vi "Send string and wait for answer or timeout.vi"(0 "System no.":i32=1 min=1 max=4 step=1, 2 "String to send":string, 3 "Attach Linefeed?":bool=TRUE, 4 "Timeout, sec":u32=60, 5 "error in":errorcluster, 12 "Stop refnum":refnum<vi>) -> (14 "String read":string, 15 "Stopped?":bool, 19 "error out":errorcluster)   [LabVIEW 2026]
doc: "Sends a string and waits until an answer has come or a timeout-condition has occured. Timeout is independent of the global communication timeout value. Sends #24 if VI was stopped. Needed by INI hexaxes and wait until finished.vi.\n\nC-887, F-206, M-8X0: INI procedure of GCS 1.0 firmware (Check with CSV?.vi. If CSV?.vi is not supported, syntax version is GCS 1.0) can be stopped with #24 since firmware version 4.0.0 (F-206) and 4.5.0 (M-8X0)."
uses:
  Communication/Global1.vi
panel:
  in  "Local stop":bool
  # "Sends a string and waits until an answer has come, a timeout \ncondition has occured, Local stop is TRUE or Stop refnum is TRUE.\n\"Timeout\" is independent of the global communication timeout \nvalue. Needed by \"INI hexaxes and wait until finished.vi\"."
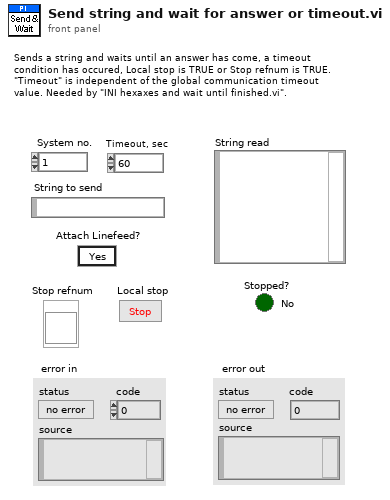
[diagram p1: front panel]
types:
  T1 = typedef "Semaphore RefNum" = refnum<k1>
  T2 = typedef "Available interfaces.ctl" = u16
  T3 = cluster{"RS232 Portnumber":i32, "Timeout":i32, "RS232 Baud rate":u32, "Interface":T2, "GPIB Bus":i32, "GPIB Address":i32, "GPIB Mode":i32}[]
  T4 = cluster{"RS232 Portnumber":i32, "Timeout":i32, "RS232 Baud rate":u32, "Interface":T2, "GPIB Bus":i32, "GPIB Address":i32, "GPIB Mode":i32}
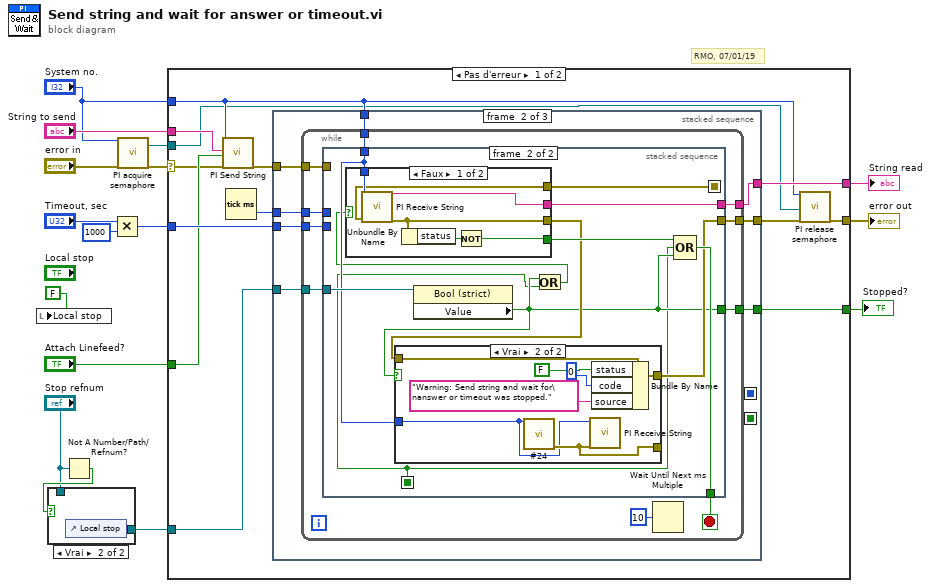
[diagram p0: block diagram]
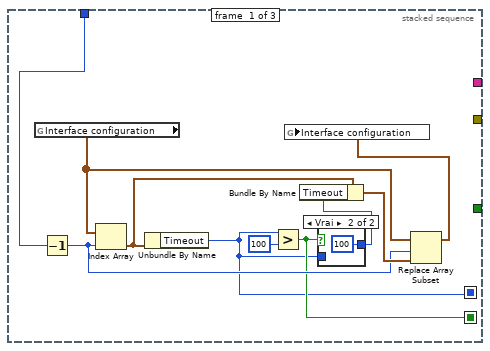
[diagram p3: hidden frame]
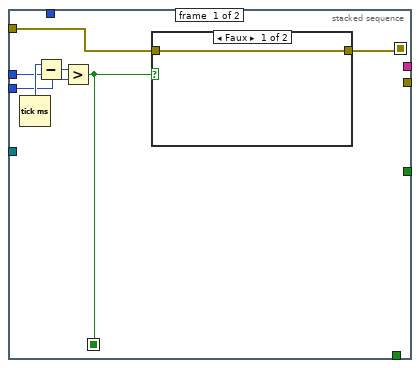
[diagram p5: hidden frame]
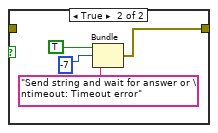
[diagram p6: hidden frame]
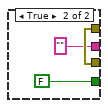
[diagram p8: hidden frame]
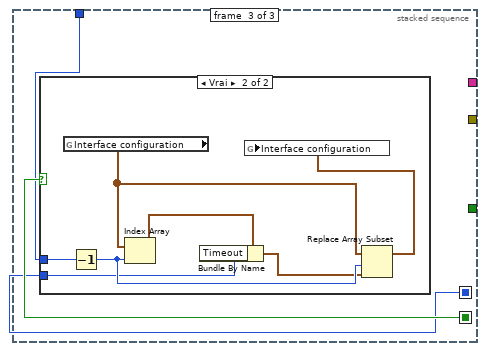
[diagram p9: hidden frame]
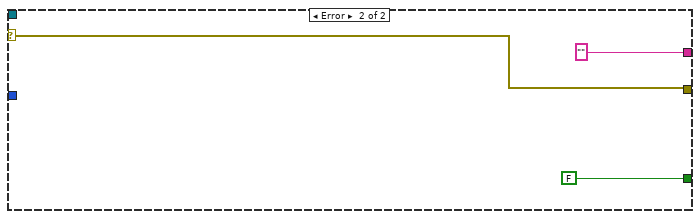
[diagram p11: hidden frame]
diagram:
  # "RMO, 07/01/19"
  n1 = local write "Local stop"(FALSE ("Local stop")) -> ()
  n2 = Not A Number/Path/Refnum?(number/path/refnum="Stop refnum") -> (NaN/Path/Refnum?=w8:bool)
  n3 = case shown="Vrai" w8 {
    tunnel: [w17 w18] -> w5
    tunnel: "Stop refnum" -> [w17 _]
    frame False {
    }
    frame True {
      n4 = control-ref of="Local stop"() -> (w18:refnum<vi>)
    }
  }
  n5 = Multiply(x="Timeout, sec", y=u32 1000) -> (x*y=w10:u32)
  n6 = call "PI acquire semaphore.vi"("System no."="System no.", "error in"="error in") -> ("semaphore out"=w1:T1, "error out"=w3:errorcluster)  [unwired: 16 out]
  n7 = case shown="Pas d'erreur" w3 {
    selector: w3 -> [w23 w112]
    tunnel: "System no." -> [w20 _]
    tunnel: w10 -> [w30 _]
    tunnel: "String to send" -> [w28 _]
    tunnel: [w21 w112] -> w15
    tunnel: [w27 "" ("String read")] -> w14
    tunnel: "Attach Linefeed?" -> [w26 _]
    tunnel: w5 -> [w25 _]
    tunnel: [w24 FALSE ("Value")] -> w6
    tunnel: w1 -> [w19 _]
    frame No Error {
      n8 = call "PI Send String.vi"("System no."=w20, "String to send"=w28, "Attach termination char.?"=w26, "error in"=w23) -> ("error out"=w31:errorcluster)  [unwired: 15 out]
      n9 = Tick Count (ms)() -> (millisecond timer value=w29:u32)
      n10 = stacked-sequence {
        seq-local: [w32 _ _] -> [_ _ w102]
        seq-local: [w33 _ _] -> [_ _ w104]
        tunnel: w20 -> [w34 w51 w103]
        tunnel: w31 -> [_ w50 _]
        tunnel: w30 -> [_ w49 _]
        tunnel: w29 -> [_ w48 _]
        tunnel: [_ w47 _] -> w22
        tunnel: [_ w46 _] -> w27
        tunnel: w25 -> [_ w45 _]
        tunnel: [_ w44 _] -> w24
        frame #0 {
          n11 = global read "Global1.vi" "Interface configuration"() -> (w38:T3)
          n12 = Decrement(x=w34) -> (x-1=w40:i32)
          n13 = Index Array(array=w38, index=w40) -> (element=w37:T4)
          n14 = Unbundle By Name(w37) -> ("Timeout"=w32:i32)
          n15 = Greater?(x=w32, y=u32 100) -> (0:w33:bool)
          n16 = case shown="Vrai" w33 {
            tunnel: [w42 100] -> w36
            tunnel: w32 -> [w42 _]
            frame False {
            }
            frame True {
            }
          }
          n17 = Bundle By Name(cluster=w37, "Timeout"=w36) -> (w41:T4)
          n18 = Replace Array Subset(array=w38, new element=w41, index=w40) -> (w39:T3)
          n19 = global write "Global1.vi" "Interface configuration"(w39) -> ()
        }
        frame #1 {
          n20 = while {
            tunnel: [w53] -> w44
            tunnel: w45 -> [w54]
            tunnel: [w55] -> w46
            tunnel: [w57] -> w47
            tunnel: w51 -> [w58]
            tunnel: w50 -> [w59]
            tunnel: w49 -> [w60]
            tunnel: w48 -> [w61]
            stop <- w56 stop-if-true
            n21 = stacked-sequence {
              seq-local: [w64 _] -> [_ w75]
              seq-local: [w62 _] -> [_ w84]
              tunnel: w61 -> [w66 _]
              tunnel: w60 -> [w65 _]
              tunnel: w59 -> [w63 _]
              tunnel: w58 -> [_ w77]
              tunnel: [_ w79] -> w57
              tunnel: [_ w82] -> w56
              tunnel: [_ w81] -> w55
              tunnel: w54 -> [_ w78]
              tunnel: [_ w76] -> w53
              frame #0 {
                n22 = Tick Count (ms)() -> (millisecond timer value=w68:u32)
                n23 = Subtract(x=w68, y=w66) -> (x-y=w67:u32)
                n24 = Greater?(x=w67, y=w65) -> (0:w64:bool)
                n25 = case shown="Faux" w64 {
                  tunnel: w63 -> [w69 _]
                  tunnel: [w69 w70] -> w62
                  frame False {
                  }
                  frame True {
                    n26 = Bundle(TRUE, -7, "Send string and wait for answer or \ntimeout: Timeout error") -> (w70:errorcluster)  [unwired: 1 out]
                  }
                }
              }
              frame #1 {
                n27 = property class="Bool (strict)"(reference=w78) -> ("Value"=w76:bool)  [unwired: 1 in, 2 out]
                n28 = Or(x=w76, y=w75) -> (x .or. y?=w74:bool)
                n29 = case shown="Faux" w74 {
                  tunnel: w77 -> [w98 _]
                  tunnel: w84 -> [w97 w101]
                  tunnel: [w96 w101] -> w80
                  tunnel: [w94 FALSE] -> w83
                  tunnel: [w93 "" ("String read")] -> w81
                  frame False {
                    n30 = call "PI Receive String.vi"("System no."=w98, "error in"=w97) -> ("String read"=w93:string, "error out"=w96:errorcluster)  [unwired: 1 in, 15 out]
                    n31 = Unbundle By Name(w96) -> ("status"=w95:bool)
                    n32 = Not(x=w95) -> (.not. x?=w94:bool)
                  }
                  frame True {
                  }
                }
                n33 = case shown="Vrai" w76 {
                  tunnel: [w85 w91] -> w79
                  tunnel: w80 -> [w85 w92]
                  tunnel: w77 -> [_ w86]
                  tunnel: [w85 w87] -> _
                  frame False {
                  }
                  frame True {
                    n34 = call "#24.vi"("System no."=w86) -> ("error out"=w87:errorcluster)  [unwired: 1 in, 17 out]
                    n35 = call "PI Receive String.vi"("System no."=w86, "error in"=w87) -> ()  [unwired: 1 in, 17 out]
                    n36 = Bundle By Name(cluster=w92, "status"=FALSE, "code"=0, "source"="Warning: Send string and wait for\nanswer or timeout was stopped.") -> (w91:errorcluster)
                  }
                }
                n37 = Compound Arithmetic op=OR(w83, w75, w76) -> (w82:bool)
              }
            }
            n38 = Wait Until Next ms Multiple(millisecond multiple=u32 10) -> ()  [unwired: 1 out]
          }
        }
        frame #2 {
          n39 = case shown="Vrai" w104 {
            tunnel: w103 -> [_ w110]
            tunnel: w102 -> [_ w105]
            frame False {
            }
            frame True {
              n40 = global read "Global1.vi" "Interface configuration"() -> (w109:T3)
              n41 = Decrement(x=w110) -> (x-1=w107:i32)
              n42 = Index Array(array=w109, index=w107) -> (element=w111:T4)
              n43 = Bundle By Name(cluster=w111, "Timeout"=w105) -> (w106:T4)
              n44 = Replace Array Subset(array=w109, new element=w106, index=w107) -> (w108:T3)
              n45 = global write "Global1.vi" "Interface configuration"(w108) -> ()
            }
          }
        }
      }
      n46 = call "PI release semaphore.vi"("System no."=w20, "semaphore"=w19, "error in"=w22) -> ("error out"=w21:errorcluster)  [unwired: 1 in, 15 out]
    }
    frame Error {
    }
  }
  "error out" <- w15
  "String read" <- w14
  "Stopped?" <- w6
